vi "Read ini file.vi"(8 "Error In":errorcluster, 11 "WS1050 1.1.lvclass":refnum<class "WS1050 1.1.lvclass">) -> (0 "Error Out":errorcluster, 3 "WS1050 1.1.lvclass Out":refnum<class "WS1050 1.1.lvclass">)   [LabVIEW 2020, in "WS1050 1.1.lvclass"]
uses:
  WS1050 1.1.lvclass
  Controls/Capacitor register.ctl
  <vilib>/Utility/config.llb/Read Key (Double).vi
  <vilib>/Utility/config.llb/NI_LVConfig.lvlib
  Toggle 7.1.lvclass
panel:
  in  "Max Beams":dbl
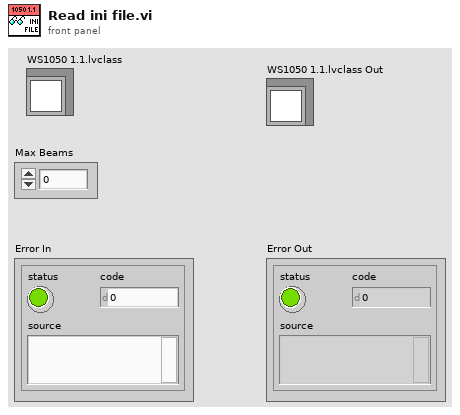
[diagram p1: front panel]
types:
  T1 = typedef "Toggle 7.1.lvclass/Capacitor register.ctl" = cluster{"Register":u32, "Beam":dbl, "Trimmers":dbl[]}
  T2 = typedef "NI_LVConfig.lvlib/Config Data RefNum.ctl" = refnum<k1>
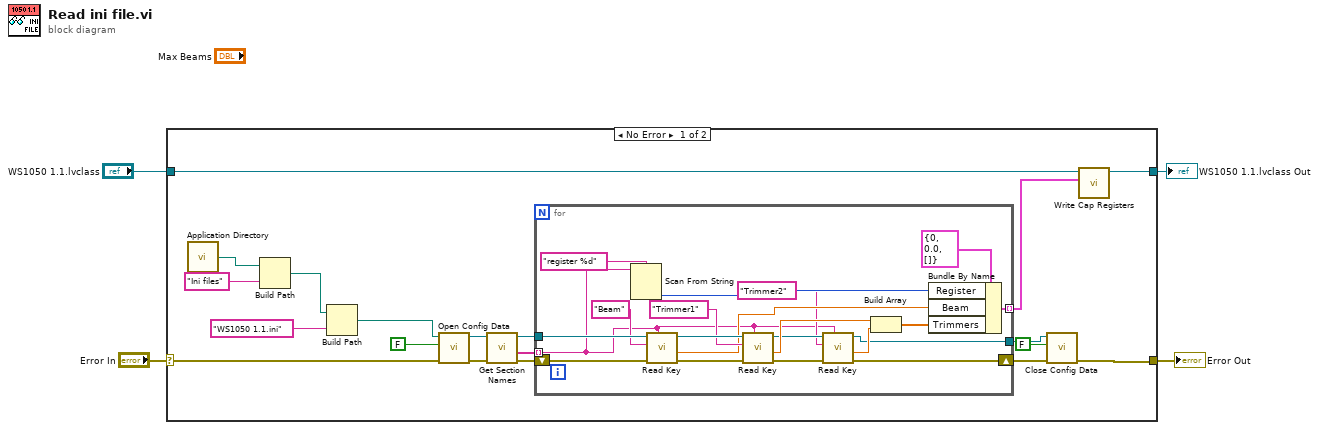
[diagram p0: block diagram]
diagram:
  n1 = case shown="No Error" "Error In" {
    selector: "Error In" -> [w20 w45]
    tunnel: [w7 w45] -> w3
    tunnel: "WS1050 1.1.lvclass" -> [w13 w44]
    tunnel: [w12 w44] -> w1
    frame No Error {
      n2 = call <vilib>:"Application Directory.vi"() -> ("Application Directory"=w23:path)
      n3 = Build Path(base path=w23, name or relative path="Ini files") -> (appended path=w5:path)
      n4 = Build Path(base path=w5, name or relative path="WS1050 1.1.ini") -> (appended path=w6:path)
      n5 = call <vilib>:"Open Config Data.vi"("error in (no error)"=w20, "create file if necessary (T)"=FALSE, "configuration file path"=w6) -> ("error out"=w18:errorcluster, "refnum"=w17:T2)  [unwired: 6 in, 1 out]
      n6 = call <vilib>:"Get Section Names.vi"("error in (no error)"=w18, "refnum"=w17) -> ("error out"=w16:errorcluster, "section names"=w15:string[], "refnum out"=w14:T2)  [unwired: 7 in]
      n7 = for {
        tunnel: w15 -> [w24] mode=indexing
        tunnel: w14 -> [w42]
        shift-right: [w27] -> w9
        shift-left: w16 -> [w43]
        tunnel: [w33] -> w11 mode=indexing
        tunnel: [w26] -> w10
        n8 = Scan From String(format string="register %d", input string=w24) -> (output 1=w36:i32)  [unwired: 3 in, 3 out]
        n9 = call-poly <vilib>:"Read Key.vi"("section"=w24, "error in (no error)"=w43, "key"="Beam", "refnum"=w42) -> ("error out"=w38:errorcluster, "value"=w35:dbl, "refnum out"=w40:T2)  [unwired: 4 in, 1 out]
        n10 = call-poly <vilib>:"Read Key.vi"("section"=w24, "error in (no error)"=w38, "key"="Trimmer1", "refnum"=w40) -> ("error out"=w32:errorcluster, "value"=w34:dbl, "refnum out"=w31:T2)  [unwired: 4 in, 1 out]
        n11 = call-poly <vilib>:"Read Key.vi"("section"=w24, "error in (no error)"=w32, "key"="Trimmer2" ("section"), "refnum"=w31) -> ("error out"=w27:errorcluster, "value"=w29:dbl, "refnum out"=w26:T2)  [unwired: 4 in, 1 out]
        n12 = Build Array(w34, w29) -> (w30:dbl[])
        n13 = Bundle By Name(cluster=T1 {"Register"=0, "Beam"=0.0, "Trimmers"=[]} ("Cap register"), "Register"=w36, "Beam"=w35, "Trimmers"=w30) -> (w33:T1)
      }
      n14 = call <vilib>:"Close Config Data.vi"("error in (no error)"=w9, "write file if changed (T)"=FALSE, "refnum"=w10) -> ("error out"=w7:errorcluster)  [unwired: 7 in, 1 out]
      n15 = call-dynamic "Write Cap Registers.vi"("Cap Registers"=w11, "Toggle 6 in"=w13) -> ("Toggle 6 out"=w12:refnum<class "WS1050 1.1.lvclass">)  [unwired: 9 in]
    }
    frame Error {
    }
  }
  "Error Out" <- w3
  "WS1050 1.1.lvclass Out" <- w1
